vi "GetStationsData.vi"(6 "access token":string, 8 "error in (no error)":errorcluster, 9 "get_favorites (F)":bool, 10 "device_id":string, 11 "token request uri":string="https://api.netatmo.com/api/getstationsdata") -> (0 "error out":errorcluster, 3 "Weather Stations Data (JSON)":string)   [LabVIEW 2020, in "Netatmo-WeatherStation.lvlib"]
uses:
  Netatmo-WeatherStation.lvlib
  <vilib>/httpClient/LabVIEWHTTPClient.lvlib
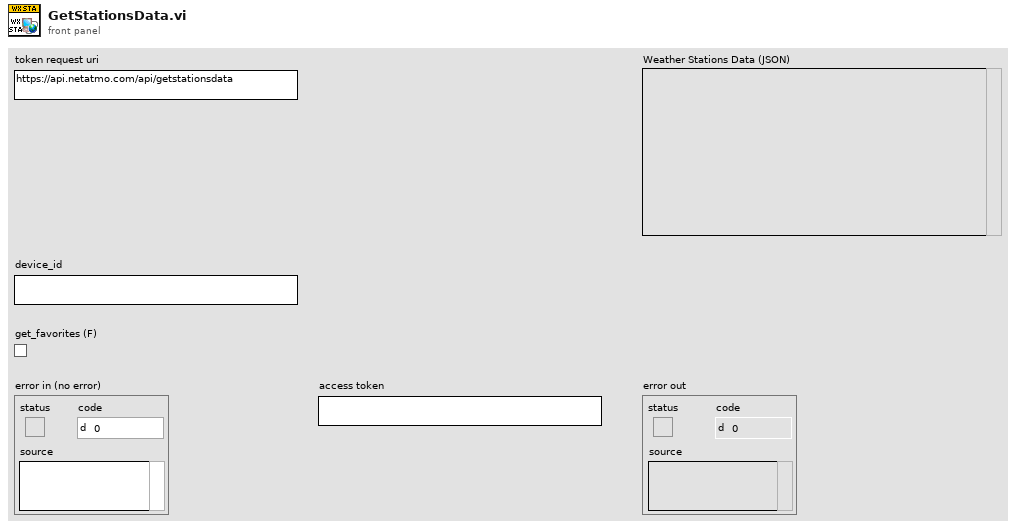
[diagram p1: front panel]
types:
  T1 = typedef "LabVIEWHTTPClient.lvlib/ClientHandle.ctl" = refnum<k1>
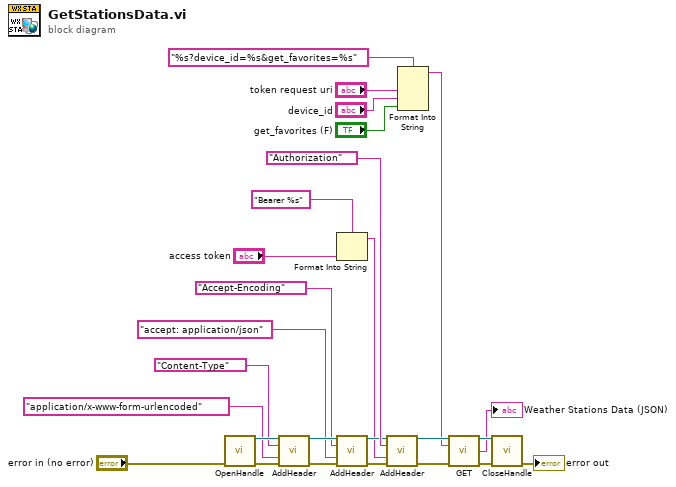
[diagram p0: block diagram]
diagram:
  n1 = call <vilib>:"OpenHandle.vi"("error in (no error)"="error in (no error)") -> ("client handle out"=w26:T1, "error out"=w20:errorcluster)  [unwired: 13 in]
  n2 = call <vilib>:"AddHeader.vi"("client handle"=w26, "header"="Content-Type", "value"="application/x-www-form-urlencoded", "error in (no error)"=w20) -> ("client handle out"=w23:T1, "error out"=w19:errorcluster)  [unwired: 10 in]
  n3 = Format Into String(format string="Bearer %s", "access token") -> (resulting string=w8:string)  [unwired: 2 in, 1 out]
  n4 = call <vilib>:"AddHeader.vi"("client handle"=w23, "header"="Accept-Encoding", "value"="accept: application/json", "error in (no error)"=w19) -> ("client handle out"=w14:T1, "error out"=w13:errorcluster)  [unwired: 10 in]
  n5 = call <vilib>:"AddHeader.vi"("client handle"=w14, "header"="Authorization", "value"=w8, "error in (no error)"=w13) -> ("client handle out"=w12:T1, "error out"=w11:errorcluster)  [unwired: 10 in]
  n6 = Format Into String(format string="%s?device_id=%s&get_favorites=%s" ("command line"), "token request uri", "device_id", "get_favorites (F)") -> (resulting string=w5:string)  [unwired: 2 in, 1 out]
  n7 = call <vilib>:"GET.vi"("client handle"=w12, "url"=w5, "error in (no error)"=w11) -> ("client handle out"=w17:T1, "body"=→"Weather Stations Data (JSON)":string, "error out"=w16:errorcluster)  [unwired: 9 in, 1 out]
  n8 = call <vilib>:"CloseHandle.vi"("client handle"=w17, "error in (no error)"=w16) -> ("error out"=→"error out":errorcluster)  [unwired: 13 in]
